vi "Read Transition.vi"(8 "error in (no error)":errorcluster, 10 "Transition Number (1: Transition 1)":i32(ring)=1 items=["Transition 1"=1, "Transition 2"=2, "Transition 3"=3, "Transition 4"=4, "Transition 5"=5, "Transition 6"=6, "Transition 7"=7, "Transition 8"=8, "Transition 9"=9, "Transition 10"=10, "Transition 11"=11, "Transition 12"=12, "Transition 13"=13, "Transition 14"=14, "Transition 15"=15, "Transition 16"=16, "Transition 17"=17, "Transition 18"=18, "Transition 19"=19, "Transition 20"=20], 11 "VISA resource name":refnum<visa-resource-name>) -> (0 "error out":errorcluster, 1 "Negative Transition Occurrence":dbl, 2 "Negative Transition Duration":dbl, 3 "VISA resource name out":refnum<visa-resource-name>, 4 "Positive Transition Occurrence":dbl, 5 "Positive Transition Duration":dbl)   [LabVIEW 2014, in "Agilent U2000 Series.lvlib"]
doc: "Returns data of a transition found on a trace.\n\nNote:\nIn case of U2040 X-Series, it is applicable for U2042XA/U2044XA/U2049XA only."
uses:
  Agilent U2000 Series.lvlib
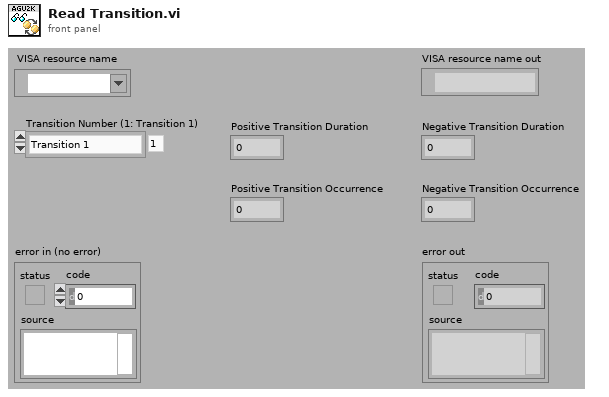
[diagram p1: front panel]
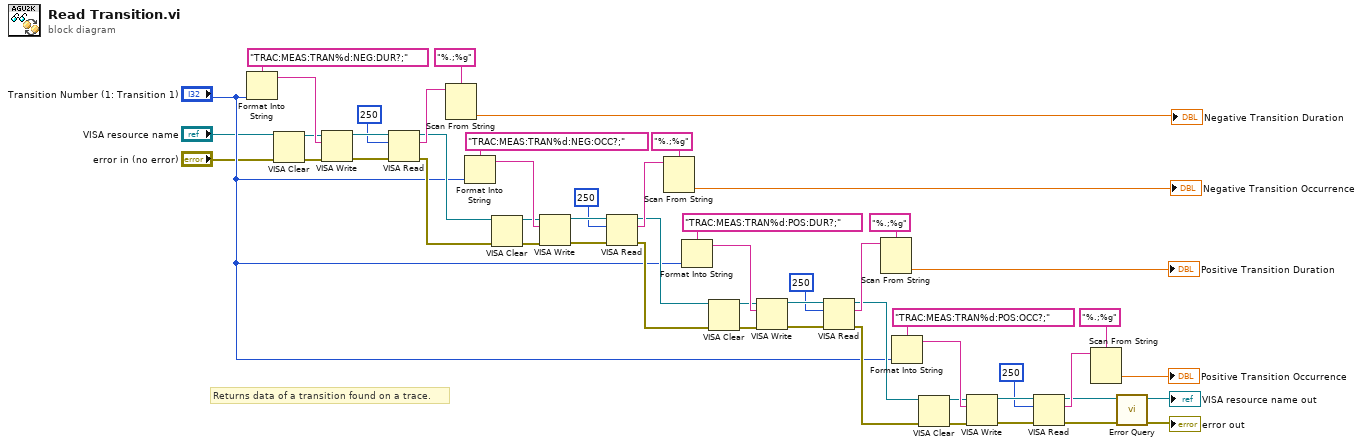
[diagram p0: block diagram]
diagram:
  # "Returns data of a transition found on a trace."
  n1 = Format Into String(format string="TRAC:MEAS:TRAN%d:NEG:DUR?;", "Transition Number (1: Transition 1)") -> (resulting string=w25:string)  [unwired: 2 in, 1 out]
  n2 = VISA Clear(VISA resource name="VISA resource name", error in (no error)="error in (no error)") -> (VISA resource name out=w19:refnum<visa-resource-name>, error out=w18:errorcluster)
  n3 = VISA Write(VISA resource name=w19, write buffer=w25, error in (no error)=w18) -> (VISA resource name out=w23:refnum<visa-resource-name>, error out=w24:errorcluster)  [unwired: 1 out]
  n4 = VISA Read(VISA resource name=w23, byte count=u32 250, error in (no error)=w24) -> (VISA resource name out=w13:refnum<visa-resource-name>, read buffer=w21:string, error out=w12:errorcluster)  [unwired: 1 out]
  n5 = Scan From String(format string="%.;%g", input string=w21) -> (output 1=→"Negative Transition Duration":dbl)  [unwired: 2 in, 4 out]
  n6 = Format Into String(format string="TRAC:MEAS:TRAN%d:NEG:OCC?;", "Transition Number (1: Transition 1)") -> (resulting string=w34:string)  [unwired: 2 in, 1 out]
  n7 = VISA Clear(VISA resource name=w13, error in (no error)=w12) -> (VISA resource name out=w28:refnum<visa-resource-name>, error out=w27:errorcluster)
  n8 = VISA Write(VISA resource name=w28, write buffer=w34, error in (no error)=w27) -> (VISA resource name out=w32:refnum<visa-resource-name>, error out=w33:errorcluster)  [unwired: 1 out]
  n9 = VISA Read(VISA resource name=w32, byte count=u32 250, error in (no error)=w33) -> (VISA resource name out=w15:refnum<visa-resource-name>, read buffer=w30:string, error out=w14:errorcluster)  [unwired: 1 out]
  n10 = Scan From String(format string="%.;%g", input string=w30) -> (output 1=→"Negative Transition Occurrence":dbl)  [unwired: 2 in, 4 out]
  n11 = Format Into String(format string="TRAC:MEAS:TRAN%d:POS:DUR?;", "Transition Number (1: Transition 1)") -> (resulting string=w43:string)  [unwired: 2 in, 1 out]
  n12 = VISA Clear(VISA resource name=w15, error in (no error)=w14) -> (VISA resource name out=w37:refnum<visa-resource-name>, error out=w36:errorcluster)
  n13 = VISA Write(VISA resource name=w37, write buffer=w43, error in (no error)=w36) -> (VISA resource name out=w41:refnum<visa-resource-name>, error out=w42:errorcluster)  [unwired: 1 out]
  n14 = VISA Read(VISA resource name=w41, byte count=u32 250, error in (no error)=w42) -> (VISA resource name out=w17:refnum<visa-resource-name>, read buffer=w39:string, error out=w16:errorcluster)  [unwired: 1 out]
  n15 = Scan From String(format string="%.;%g", input string=w39) -> (output 1=→"Positive Transition Duration":dbl)  [unwired: 2 in, 4 out]
  n16 = Format Into String(format string="TRAC:MEAS:TRAN%d:POS:OCC?;", "Transition Number (1: Transition 1)") -> (resulting string=w52:string)  [unwired: 2 in, 1 out]
  n17 = VISA Clear(VISA resource name=w17, error in (no error)=w16) -> (VISA resource name out=w46:refnum<visa-resource-name>, error out=w45:errorcluster)
  n18 = VISA Write(VISA resource name=w46, write buffer=w52, error in (no error)=w45) -> (VISA resource name out=w50:refnum<visa-resource-name>, error out=w51:errorcluster)  [unwired: 1 out]
  n19 = VISA Read(VISA resource name=w50, byte count=u32 250, error in (no error)=w51) -> (VISA resource name out=w4:refnum<visa-resource-name>, read buffer=w48:string, error out=w3:errorcluster)  [unwired: 1 out]
  n20 = Scan From String(format string="%.;%g", input string=w48) -> (output 1=→"Positive Transition Occurrence":dbl)  [unwired: 2 in, 4 out]
  n21 = call "Error Query.vi"("error in (no error)"=w3, "VISA resource name"=w4) -> ("error out"=→"error out":errorcluster, "VISA resource name out"=→"VISA resource name out":refnum<visa-resource-name>)  [unwired: 8 out]
